vi "Parse Data Replay Control.vi"(7 "Controls":T1[](array[typedef]), 10 "Control Name":string="RPMThreshold", 11 "LUT in":variant) -> (3 "LUT out":variant)   [LabVIEW 2011, in "Engine Sim System Explorer.lvlib"]
uses:
  Engine Sim System Explorer.lvlib
  <userlib>/_FPGA Interface Advanced Tools/FPGA Bitfile Utility/TypeDefs/Scalar Register.ctl
  <vilib>/regexp/Match Regular Expression.xnode
  <userlib>/_FPGA Interface Advanced Tools/FPGA Bitfile Utility/FPGA Bitfile Utility.lvlib
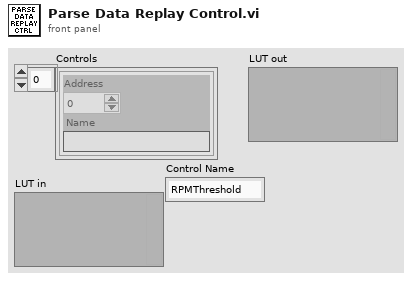
[diagram p1: front panel]
types:
  T1 = typedef "FPGA Bitfile Utility.lvlib/Scalar Register.ctl" = cluster{"Address":u32, "Name":string}
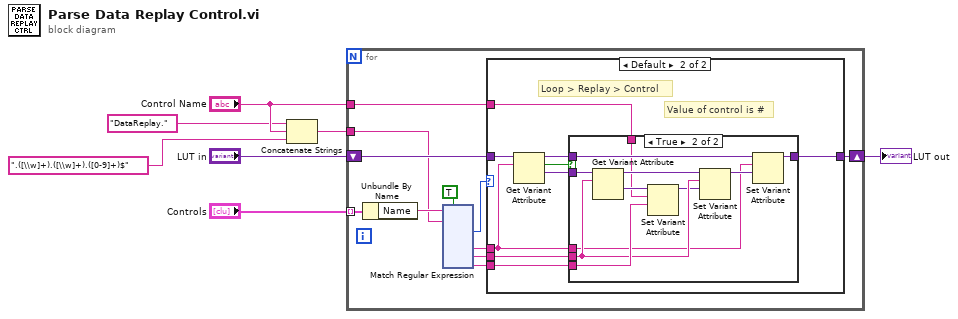
[diagram p0: block diagram]
diagram:
  n1 = Concatenate Strings("DataReplay." ("regular expression"), "Control Name", ".([\\w]+).([\\w]+).([0-9]+)$" ("regular expression")) -> (w1:string)
  n2 = for {
    tunnel: "Controls" -> [w16] mode=indexing
    shift-right: [w13] -> w7
    shift-left: "LUT in" -> [w15]
    tunnel: "Control Name" -> [w9]
    tunnel: w1 -> [w8]
    n3 = Unbundle By Name(w16) -> ("Name"=w17:string)
    n4 = xnode "Match Regular Expression"("input string"=w17, "regular expression"=w8, "ignore case? (F)"=TRUE) -> ("offset past match"=w14:i32, "submatch 1"=w12:string, "submatch 2"=w11:string, "submatch 3"=w10:string)  [unwired: 3 in, 4 out]
    n5 = case shown="Default" w14 {
      tunnel: w15 -> [w19 w28]
      tunnel: [w19 w22] -> w13
      tunnel: w12 -> [_ w24]
      tunnel: w11 -> [_ w25]
      tunnel: w10 -> [_ w26]
      tunnel: w9 -> [_ w21]
      frame -1 {
      }
      frame Default {
        # "Value of control is #"
        # "Loop > Replay > Control"
        n6 = Get Variant Attribute(Variant=w28, name=w24) -> (duplicate Variant=w23:variant, found=w20:bool, value=w27:variant)  [unwired: 2 in, 1 out]
        n7 = case shown="True" w20 {
          tunnel: w27 -> [_ w40]
          tunnel: w26 -> [_ w38]
          tunnel: w25 -> [_ w36]
          tunnel: w24 -> [_ w33]
          tunnel: w23 -> [w29 w32]
          tunnel: [w29 w31] -> w22
          tunnel: w21 -> [_ w30]
          frame False {
            # "The loop this claims was not previously detected"
          }
          frame True {
            n8 = Get Variant Attribute(Variant=w40, name=w36) -> (duplicate Variant=w37:variant, value=w39:variant)  [unwired: 2 in, 2 out]
            n9 = Set Variant Attribute(Variant=w39, name=w30, value=w38) -> (Variant out=w35:variant)  [unwired: 1 in, 2 out]
            n10 = Set Variant Attribute(Variant=w37, name=w36, value=w35) -> (Variant out=w34:variant)  [unwired: 1 in, 2 out]
            n11 = Set Variant Attribute(Variant=w32, name=w33, value=w34) -> (Variant out=w31:variant)  [unwired: 1 in, 2 out]
          }
        }
      }
    }
  }
  "LUT out" <- w7
